vi "Stop ZeroMQ VIs.vi"(8 "error in (no error)":errorcluster, 11 "Header content in":refnum<class "Header content.lvclass">) -> (0 "error out":errorcluster, 3 "Header content out":refnum<class "Header content.lvclass">)   [LabVIEW 2018, in "Header content.lvclass"]
uses:
  Header content.lvclass
  Header content.lvclass/Header content.ctl
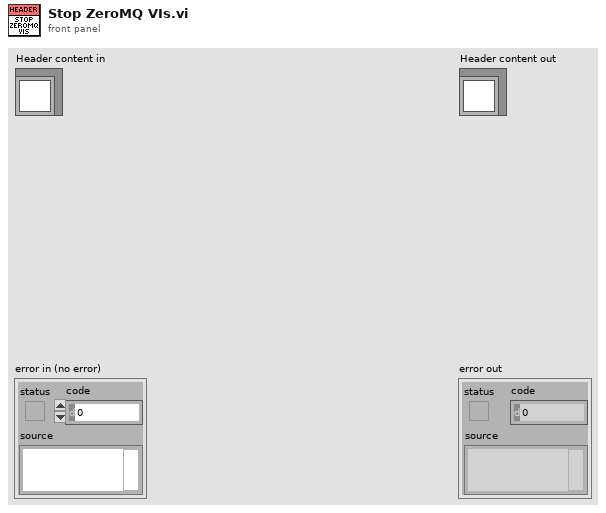
[diagram p1: front panel]
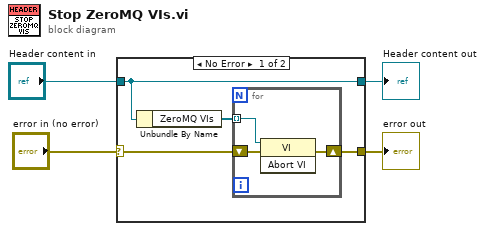
[diagram p0: block diagram]
diagram:
  n1 = case shown="No Error" "error in (no error)" {
    selector: "error in (no error)" -> [w7 w13]
    tunnel: [w6 w13] -> w3
    tunnel: [w8 w12] -> w1
    tunnel: "Header content in" -> [w8 w12]
    frame No Error {
      n2 = Unbundle By Name(w8) -> ("ZeroMQ VIs"=w5:refnum<vi>[])
      n3 = for {
        shift-right: [w10] -> w6
        shift-left: w7 -> [w11]
        tunnel: w5 -> [w9] mode=indexing
        n4 = invoke class="VI" method="Abort VI"(reference=w9, error in=w11) -> (error out=w10:errorcluster)  [unwired: 1 in, 2 out]
      }
    }
    frame Error {
    }
  }
  "error out" <- w3
  "Header content out" <- w1
